vi "Thread@SubThreadEnd__Parameter.vi"(1 "ParamterIn":string) -> (0 "ParamterOut":string)   [LabVIEW 2019]
uses:
  MainFrame/Global.vi
panel:
  in  "Thread Label":string(combo)
  in  "Confirm":bool
  # "Thread@SubThreadEnd $SubName"
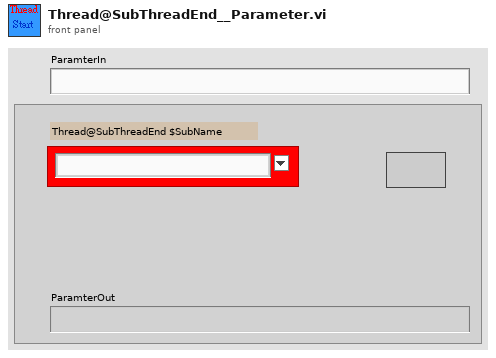
[diagram p1: front panel]
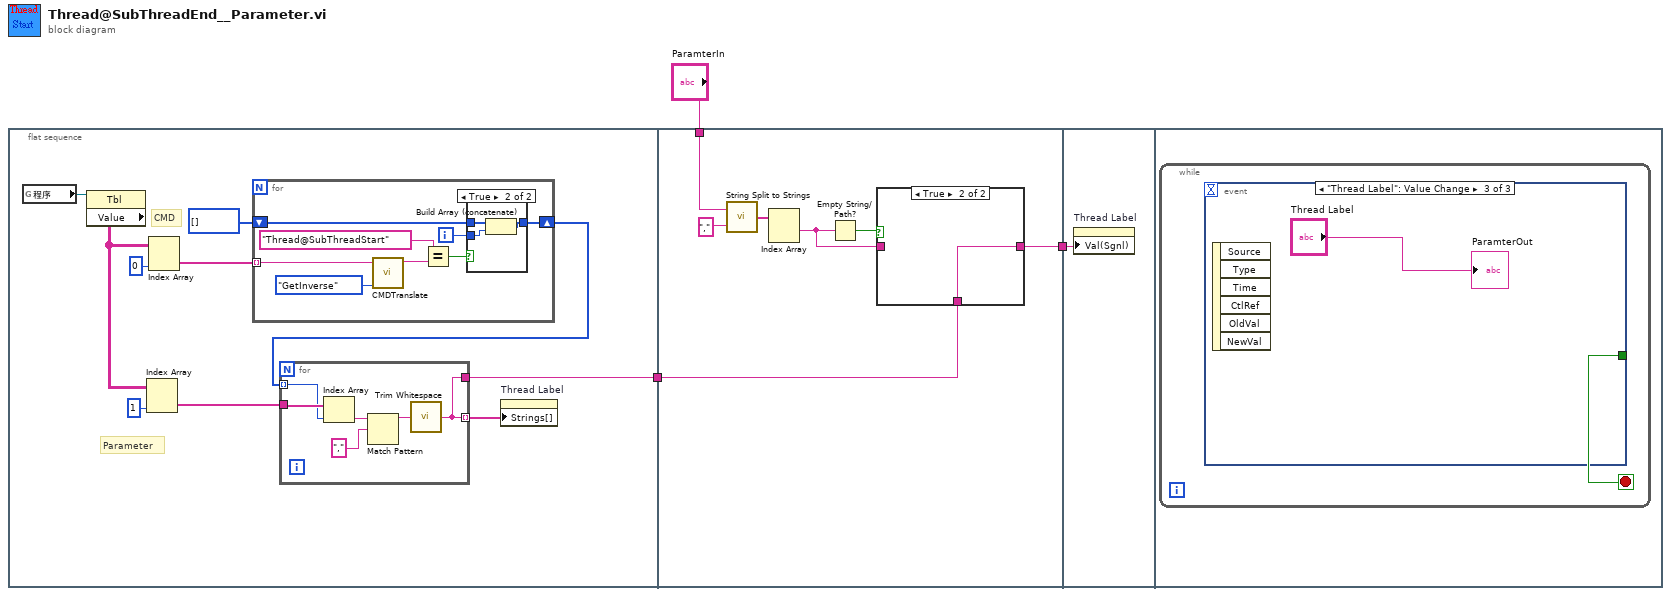
[diagram p0: block diagram]
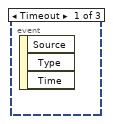
[diagram p4: hidden frame]
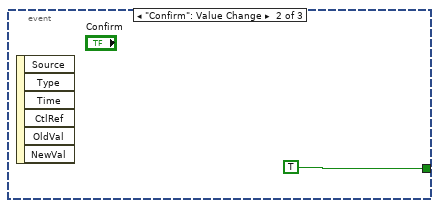
[diagram p5: hidden frame]
diagram:
  n1 = flat-sequence {
    tunnel: [w4] -> w1
    tunnel: "ParamterIn" -> [w36]
    tunnel: [w33] -> w2
    tunnel: w1 -> [w32]
    tunnel: w2 -> [w41]
    frame #0 {
      # "Parameter"
      # "CMD"
      n2 = global read "Global.vi" "程序"() -> (w13:refnum<vi>)
      n3 = property class="Tbl"(reference=w13) -> ("Value"=w10:string[][])  [unwired: 1 in, 2 out]
      n4 = Index Array(array=w10, index (col)=1 ("index (row)")) -> (element=w7:string[])  [unwired: 1 in]
      n5 = Index Array(array=w10, index (col)=0 ("index (row)")) -> (element=w9:string[])  [unwired: 1 in]
      n6 = for {
        tunnel: w9 -> [w26] mode=indexing
        shift-right: [w20] -> w6
        shift-left: i32[] [] -> [w22]
        i -> [w21]
        n7 = call "CMDTranslate.vi"("OP"=enum16{"Init", "Set", "Get", "GetInverse"}."GetInverse", "CMDIn"=w26) -> ("CMDOut"=w25:string)  [unwired: 9 in]
        n8 = Equal?(x="Thread@SubThreadStart", y=w25) -> (x = y?=w23:bool)
        n9 = case shown="True" w23 {
          tunnel: w22 -> [w28 w31]
          tunnel: w21 -> [_ w30]
          tunnel: [w28 w29] -> w20
          frame False {
          }
          frame True {
            n10 = Build Array (concatenate)(w31, w30) -> (w29:i32[])
          }
        }
      }
      n11 = for {
        tunnel: w7 -> [w19]
        tunnel: w6 -> [w18] mode=indexing
        tunnel: [w15] -> w5 mode=indexing
        tunnel: [w15] -> w4
        n12 = Index Array(array=w19, index=w18) -> (element=w17:string)
        n13 = Match Pattern(string=w17, regular expression=",") -> (before substring=w14:string)  [unwired: 1 in, 3 out]
        n14 = call <vilib>:"Trim Whitespace.vi"("string"=w14) -> ("trimmed string"=w15:string)  [unwired: 1 in]
      }
      n15 = property on="Thread Label" class="CmbBox"("Strings[]"=w5) -> ()  [unwired: 2 in, 2 out]
    }
    frame #1 {
      n16 = call "String Split to Strings.vi"("search string/char (-)"=",", "String"=w36) -> ("Array"=w38:string[])
      n17 = Index Array(array=w38) -> (element #1=w34:string)  [unwired: 2 in, 1 out]
      n18 = Empty String/Path?(string/path=w34) -> (empty?=w35:bool)
      n19 = case shown="True" w35 {
        tunnel: w34 -> [w39 _]
        tunnel: [w39 w40] -> w33
        tunnel: w32 -> [_ w40]
        frame False {
        }
        frame True {
        }
      }
    }
    frame #2 {
      n20 = property on="Thread Label" class="CmbBox"("Val(Sgnl)"=w41) -> ()  [unwired: 2 in, 2 out]
    }
    frame #3 {
      n21 = while {
        stop <- w42 stop-if-true
        n22 = event shown="[2] \"Thread Label\": Value Change" {
          selector: _ -> [_ _ _]
          dyn-events: _ -> [_ _ _]
          timeout: _ -> [_ _ _]
          tunnel: [_ TRUE _] -> w42
          event Timeout {
            n23 = event-data() -> ()  [unwired: 1 in, 3 out]
          }
          event "Confirm": Value Change {
            n24 = event-data() -> ()  [unwired: 1 in, 6 out]
          }
          event "Thread Label": Value Change {
            n25 = event-data() -> ()  [unwired: 1 in, 6 out]
            "ParamterOut" <- "Thread Label"
          }
        }
      }
    }
  }
